vi "Waveform Generation.vi"(11 "Cluster":T1) -> (1 "Output Y Values":dbl[](array[numeric]), 3 "Waveform":waveform(dbl))   [LabVIEW 2014]
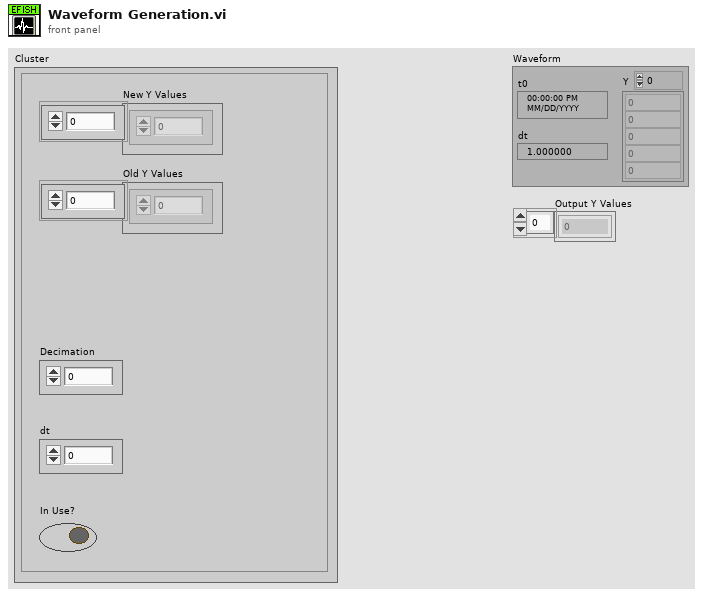
[diagram p1: front panel]
types:
  T1 = cluster{"New Y Values":dbl[], "Old Y Values":dbl[], "Decimation":i32, "dt":dbl, "In Use?":bool}
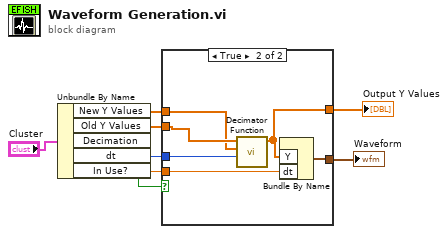
[diagram p0: block diagram]
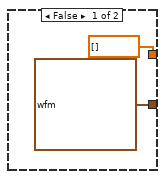
[diagram p2: hidden frame]
diagram:
  n1 = Unbundle By Name("Cluster") -> ("New Y Values"=w7:dbl[], "Old Y Values"=w6:dbl[], "Decimation"=w5:i32, "dt"=w3:dbl, "In Use?"=w4:bool)
  n2 = case shown="True" w4 {
    tunnel: w6 -> [_ w13]
    tunnel: w7 -> [_ w12]
    tunnel: w5 -> [_ w16]
    tunnel: w3 -> [_ w11]
    tunnel: [waveform(dbl) {"t0"=timestamp(0 s since 1904-01-01), "dt"=1.0, "Y"=[]} w15] -> w2
    tunnel: [dbl[] [] ("Output Y Values") w14] -> w1
    frame False {
    }
    frame True {
      n3 = call "Decimator Function.vi"("Decimation #"=w16, "Input Y values New"=w12, "Input Y values Old"=w13) -> ("Output Y Values"=w14:dbl[])  [unwired: 8 in]
      n4 = Bundle By Name("Y"=w14, "dt"=w11) -> (w15:waveform(dbl))  [unwired: 1 in]
    }
  }
  "Waveform" <- w2
  "Output Y Values" <- w1
